vi "Get Provider Name.vi"(8 "error in (no error)":errorcluster, 11 "ADODB in":refnum<class "ADODB.lvclass">) -> (0 "error out":errorcluster, 2 "Provider Name":string, 3 "ADODB out":refnum<class "ADODB.lvclass">)   [LabVIEW 2020, in "ADODB.lvlib" / "ADODB.lvclass"]
uses:
  ADODB.lvclass
  ADODB.lvclass/ADODB.ctl
  <vilib>/addons/database/NI_Database_API.lvlib
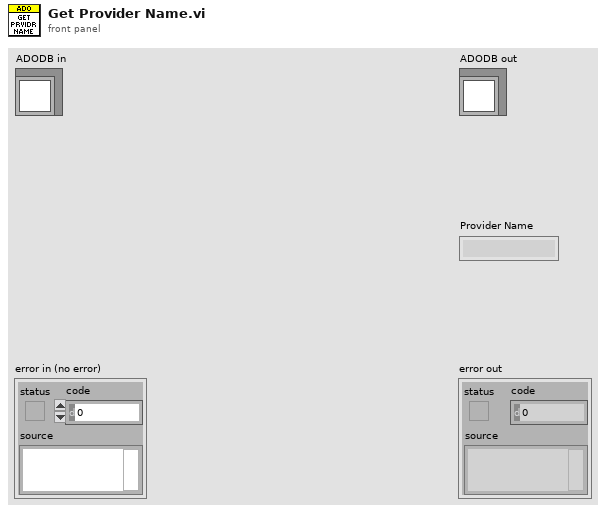
[diagram p1: front panel]
types:
  T1 = typedef "NI_Database_API.lvlib/Conn ObjectReference.ctl" = refnum<k1>
  T2 = typedef "NI_Database_API.lvlib/Conn DataMembers.ctl" = cluster{"ADODB._Connection":refnum<k7>, "recordset objects":i32, "command objects":i32}
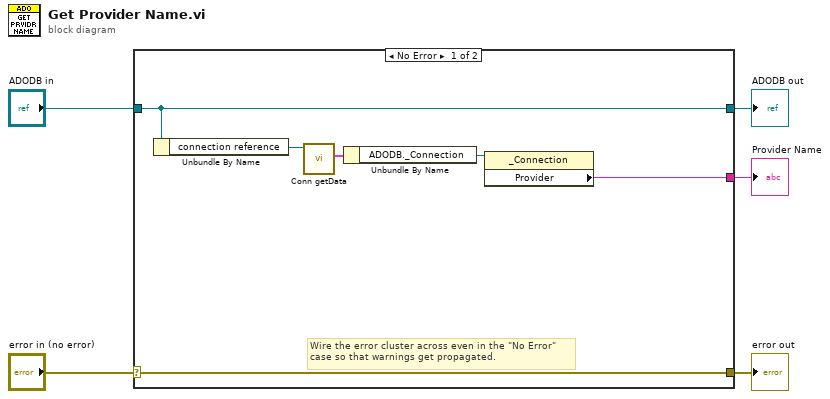
[diagram p0: block diagram]
diagram:
  n1 = case shown="No Error" "error in (no error)" {
    selector: "error in (no error)" -> [w11 w13]
    tunnel: [w11 w13] -> w4
    tunnel: [w10 w12] -> w2
    tunnel: "ADODB in" -> [w10 w12]
    tunnel: [w6 _] -> w1
    frame No Error {
      # "Wire the error cluster across even in the \"No Error\"\ncase so that warnings get propagated."
      n2 = Unbundle By Name(w10) -> ("connection reference"=w9:T1)
      n3 = call <vilib>:"Conn getData.vi"("connection reference"=w9) -> ("data"=w8:T2)  [unwired: 3 in, 3 out]
      n4 = Unbundle By Name(w8) -> ("ADODB._Connection"=w7:refnum<k7>)
      n5 = property class="_Connection"(reference=w7) -> ("Provider"=w6:string)  [unwired: 1 in, 2 out]
    }
    frame Error {
    }
  }
  "error out" <- w4
  "ADODB out" <- w2
  "Provider Name" <- w1
